vi "Protocol Main.vi"() -> ()   [LabVIEW 2014]
doc: "Diese Vorlage beschreibt das Design \"Handler für Nachrichten-Queues\".\n\nDie Schleife zur Ereignisbehandlung erzeugt Nachrichten basierend auf Benutzereingaben.\n\nDie Schleife zur Nachrichtenbehandlung verarbeitet Nachrichten, die von der Ereignisschleife oder anderen Nachrichten erzeugt wurden. Die Nachrichten sind String-Werte. Neue Nachrichten können also einfach der Case-Struktur der Nachrichtenschleife hinzugefügt werden. Der Nachrichten-Cluster kann auch einen optionalen Wert für Nachrichtendaten enthalten. Dabei handelt es sich um einen Variant, der in beliebige nachrichtenspezifische Daten umgewandelt werden kann."
uses:
  controls/ProtocolT.ctl
  controls/ProtocolEntry.ctl
  controls/MyQH UI Data.ctl
  support/Message Queue/Enqueue Message (Single).vi
  support/Message Queue/Enqueue Message (Array).vi
  <vilib>/Utility/error.llb/Error Cluster From Error Code.vi
  <vilib>/ErrorRing/Error Ring.xnode
  support/Message Queue/MyQH Message Queue.lvlib
  support/User Event - Stop/MyQH User Event - Stop.lvlib
panel:
  in  "Load":bool
  in  "Save":bool
  in  "ProtocolT":T1 {"Zeitstempel" format=" %<%X %x>T"}
  out "Anzeige <Ersetzen>":string
  in  "Remove Entry":bool
  in  "Add Entry":bool
  in  "Beenden":bool
  # "Titel"
  # "Eintrag"
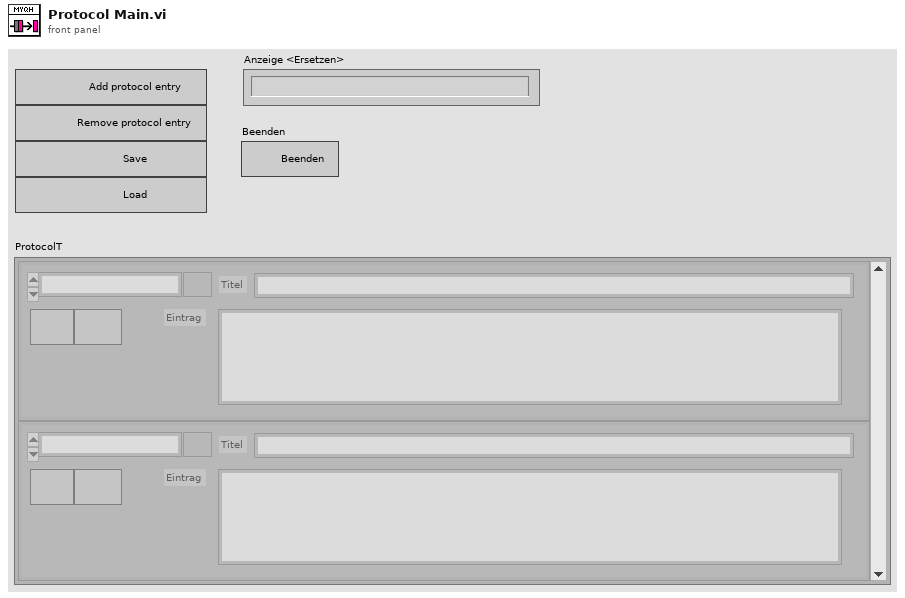
[diagram p1: front panel]
types:
  T1 = typedef "ProtocolT.ctl" = T2[]
  T2 = typedef "ProtocolEntry.ctl" = cluster{"Zeitstempel":timestamp, "String":string, "Abbrechen-Schaltfläche":bool, "Optionen-Schaltfläche":bool, "String 2":string}
  T3 = typedef "MyQH UI Data.ctl" = cluster{"Boolesch <Ersetzen>":bool, "String <Ersetzen>":string, "Numerisch <Ersetzen>":dbl, "Etwas tun (Ref.)":refnum<vi>, "Etwas anderes tun (Ref.)":refnum<vi>, "Datenanzeige (Ref.)":refnum<vi>, "Beenden-Schaltfl. (Ref.)":refnum<vi>, "Cluster":cluster{"VI Referenz":refnum<vi>}, "Arr Referenz":refnum<vi>, "Cluster Referenz":refnum<vi>, "ProtocolT":T1, "ProtocolEntryT":T2}
  T4 = cluster{"Status":bool, "Code":i32, "Quelle":string}
  T5 = typedef "MyQH Message Queue.lvlib/All Message Queues.ctl" = cluster{"UI":refnum<queue>}
  T6 = enum16{"big-endian, network order", "native, host order", "little-endian"}
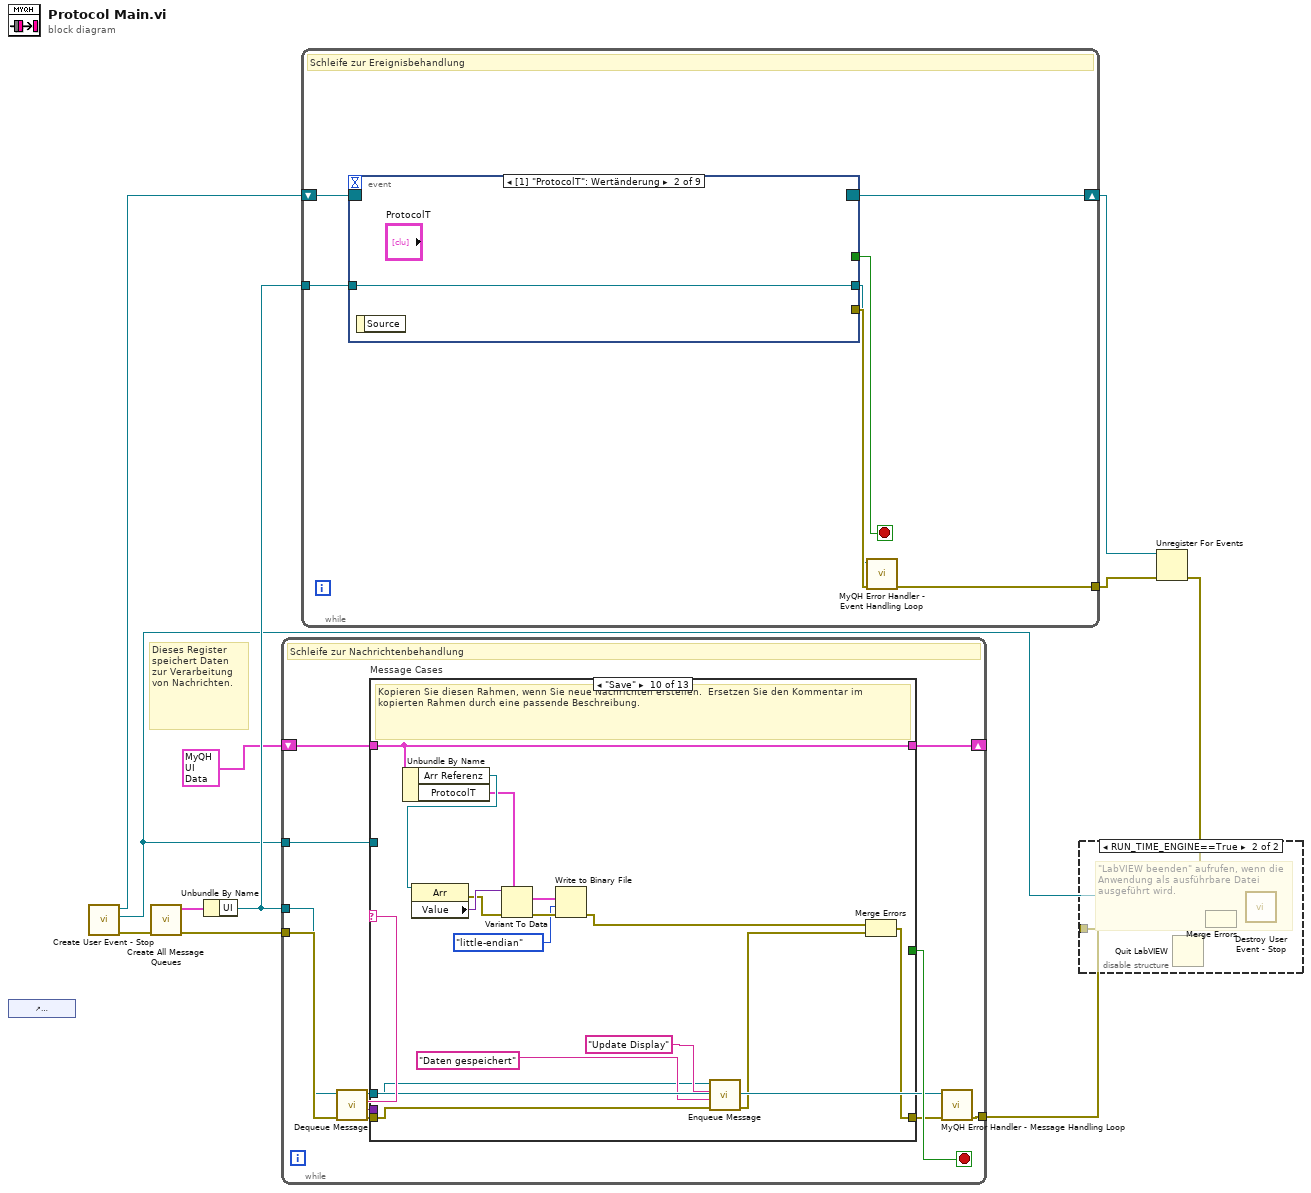
[diagram p0: block diagram]
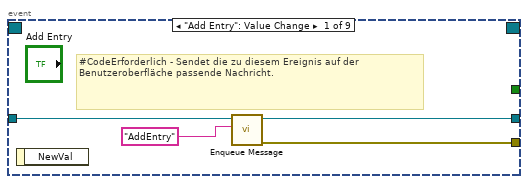
[diagram p3: hidden frame]
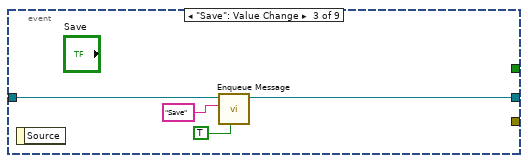
[diagram p4: hidden frame]
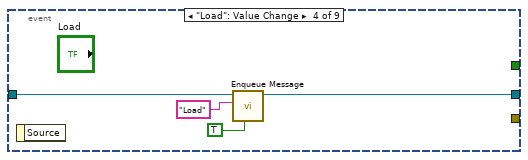
[diagram p5: hidden frame]
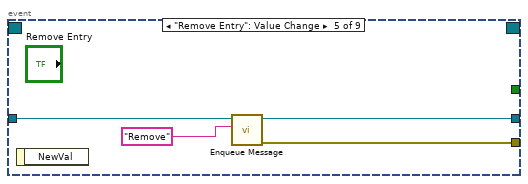
[diagram p6: hidden frame]
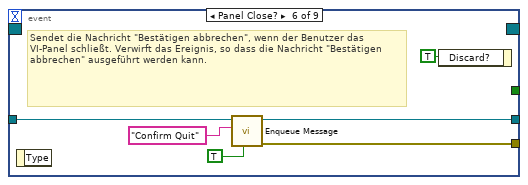
[diagram p7: hidden frame]
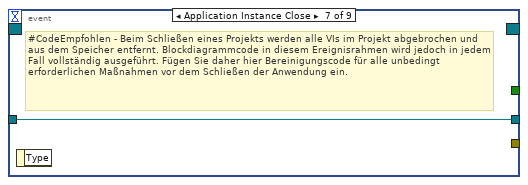
[diagram p8: hidden frame]
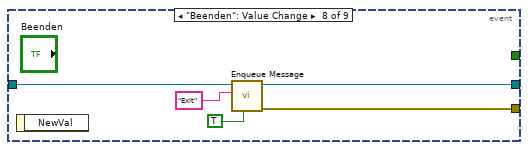
[diagram p9: hidden frame]
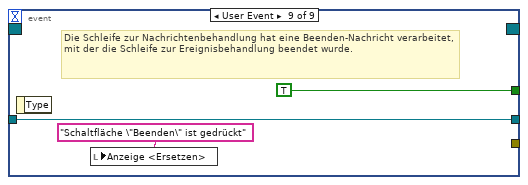
[diagram p10: hidden frame]
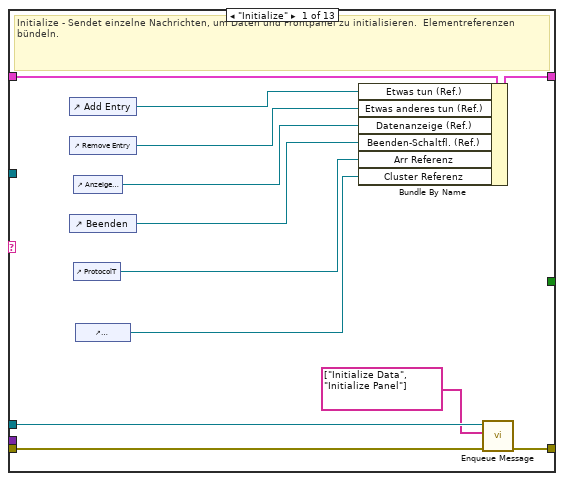
[diagram p11: hidden frame]
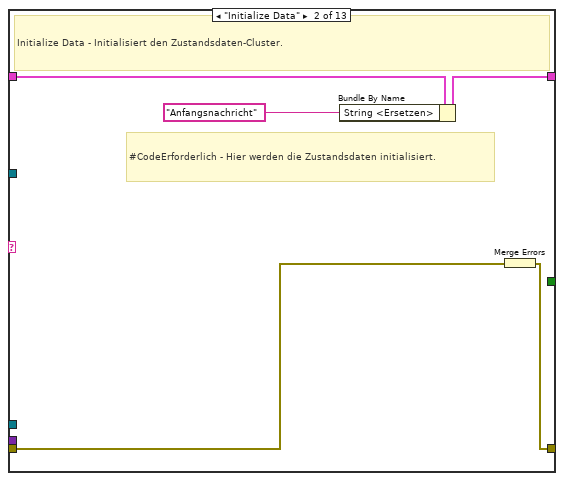
[diagram p12: hidden frame]
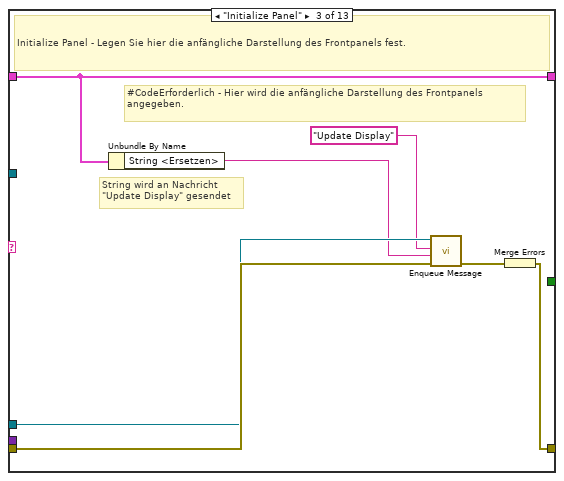
[diagram p13: hidden frame]
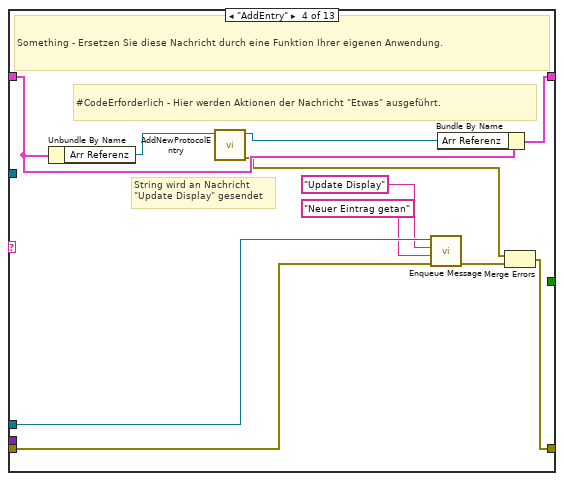
[diagram p14: hidden frame]
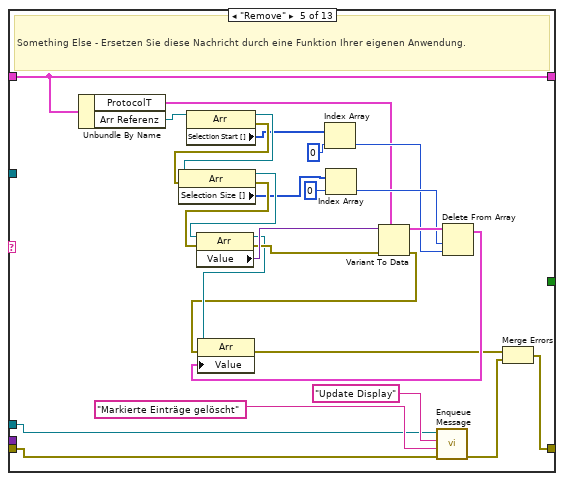
[diagram p15: hidden frame]
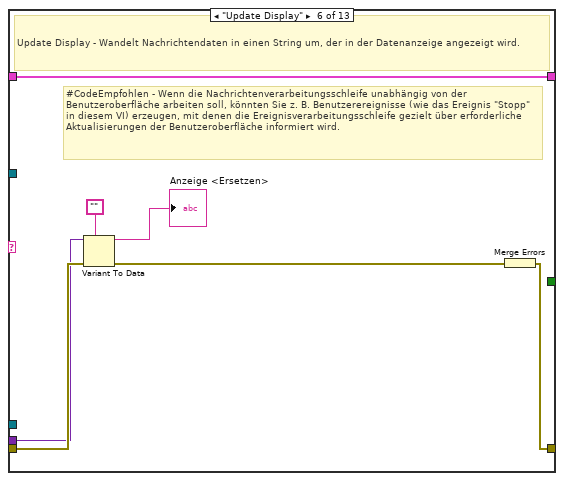
[diagram p16: hidden frame]
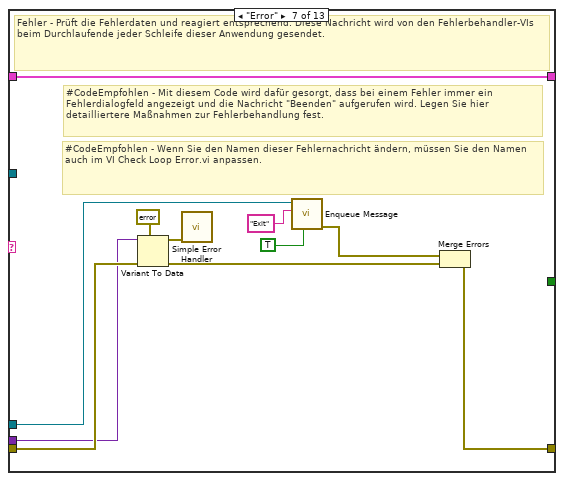
[diagram p17: hidden frame]
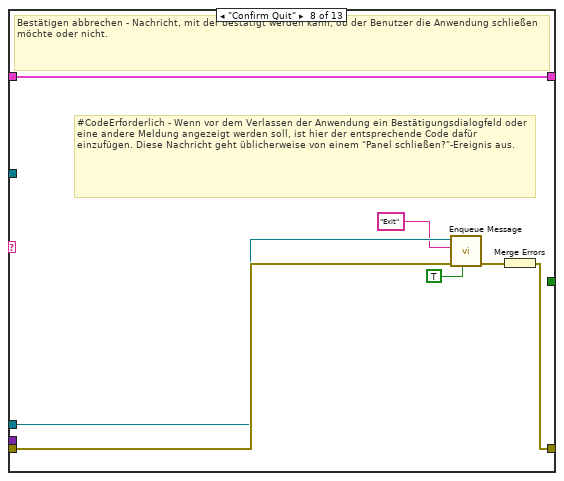
[diagram p18: hidden frame]
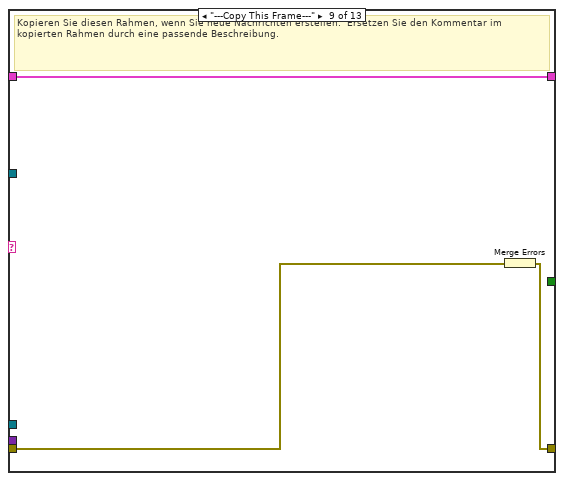
[diagram p19: hidden frame]
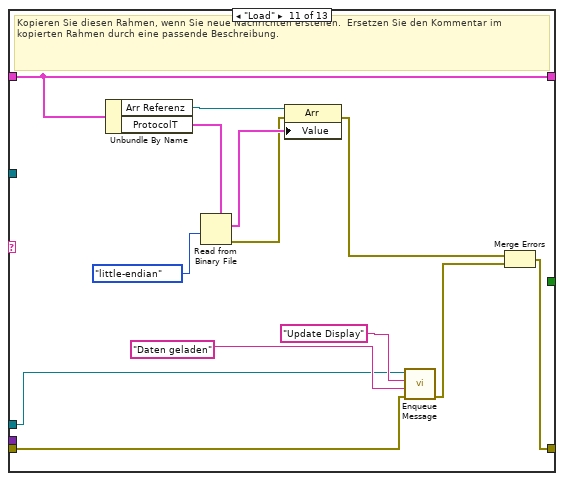
[diagram p20: hidden frame]
diagram:
  # "Dieses Register speichert Daten zur Verarbeitung von Nachrichten."
  n1 = control-ref of="Abbrechen-Schaltfläche"() -> ()  [unwired: 1 out]
  n2 = call "Create User Event - Stop.vi"() -> ("error out"=w8:T4, "Benutzerereignis - Stopp"=w6:refnum<user-event>, "Stoppereignisregistrierung (Referenz)"=w9:refnum<event-registration>)  [unwired: 9 in]
  n3 = call "Create All Message Queues.vi"("error in (no error)"=w8) -> ("error out"=w13:T4, "Nachrichten-Queues (Ausgang)"=w12:T5)  [unwired: 9 in]
  n4 = Unbundle By Name(w12) -> ("UI"=w10:refnum<queue>)
  n5 = while {
    tunnel: w10 -> [w17]
    shift-right: [w24] -> _
    shift-left: T3 {"Boolesch <Ersetzen>"=FALSE, "String <Ersetzen>"="", "Numerisch <Ersetzen>"=0.0, "Etwas tun (Ref.)"=refnum, "Etwas anderes tun (Ref.)"=refnum, "Datenanzeige (Ref.)"=refnum, "Beenden-Schaltfl. (Ref.)"=refnum, "Cluster"={"VI Referenz"=refnum}, "Arr Referenz"=refnum, "Cluster Referenz"=refnum, "ProtocolT"=[], "ProtocolEntryT"={"Zeitstempel"=timestamp(0 s since 1904-01-01), "String"="", "Abbrechen-Schaltfläche"=FALSE, "Optionen-Schaltfläche"=FALSE, "String 2"=""}} ("Data Cluster") -> [w25]
    tunnel: w6 -> [w22]
    tunnel: w13 -> [w21]
    tunnel: [w15] -> w11
    stop <- w23 stop-if-true
    # "Schleife zur Nachrichtenbehandlung"
    n6 = call "Dequeue Message.vi"("error in (no error)"=w21, "Nachrichten-Queue"=w17) -> ("error out"=w20:T4, "Nachrichtendaten"=w18:variant, "Nachricht"=w19:string, "Nachrichten-Queue (Kopie)"=w16:refnum<queue>)  [unwired: 6 in]
    n7 = case "Message Cases" shown="\"Save\"" w19 {
      selector: w19 -> [_ _ _ _ _ _ _ _ _ _ _ _ w151]
      tunnel: w16 -> [w35 _ w46 w57 w63 _ w96 w107 _ w116 w132 w150 _]
      tunnel: w20 -> [w36 w42 w47 w59 w62 w91 w104 w111 w114 w117 w130 w145 _]
      tunnel: [w37 w38 w48 w60 w86 w92 w97 w109 w112 w129 w142 w146 w152] -> w14
      tunnel: w25 -> [w34 w41 w49 w52 w67 w93 w103 w110 w113 w128 w140 w149 w153]
      tunnel: [w33 w40 w49 w51 w67 w93 w103 w110 w113 w128 w140 w149 w153] -> w24
      tunnel: [_ _ _ _ _ _ _ _ _ _ _ TRUE _] -> w23
      tunnel: w18 -> [_ _ _ _ _ w90 w102 _ _ _ _ _ _]
      tunnel: w22 -> [_ _ _ _ _ _ _ _ _ _ _ w144 _]
      frame "Initialize" {
        # "Initialize - Sendet einzelne Nachrichten, um Daten und Frontpanel zu initialisieren.  Elementreferenzen bündeln."
        n8 = control-ref of="Add Entry"() -> (w32:refnum<vi>)
        n9 = control-ref of="Remove Entry"() -> (w31:refnum<vi>)
        n10 = control-ref of="Beenden"() -> (w29:refnum<vi>)
        n11 = control-ref of="Anzeige <Ersetzen>"() -> (w30:refnum<vi>)
        n12 = control-ref of="ProtocolT"() -> (w27:refnum<vi>)
        n13 = control-ref of="ProtocolEntryT"() -> (w26:refnum<vi>)
        n14 = Bundle By Name(cluster=w34, "Etwas tun (Ref.)"=w32, "Etwas anderes tun (Ref.)"=w31, "Datenanzeige (Ref.)"=w30, "Beenden-Schaltfl. (Ref.)"=w29, "Arr Referenz"=w27, "Cluster Referenz"=w26) -> (w33:T3)
        n15 = call-poly "Enqueue Message.vi"("error in (no error)"=w36, "Nachrichten-Array"=string[] ["Initialize Data", "Initialize Panel"], "Nachrichten-Queue"=w35) -> ("error out"=w37:T4)  [unwired: 7 in, 1 out]
      }
      frame "Initialize Data" {
        # "#CodeErforderlich - Hier werden die Zustandsdaten initialisiert."
        # "Initialize Data - Initialisiert den Zustandsdaten-Cluster."
        n16 = Bundle By Name(cluster=w41, "String <Ersetzen>"="Anfangsnachricht" ("Initial Message")) -> (w40:T3)
        n17 = Merge Errors(w42) -> (w38:errorcluster)
      }
      frame "Initialize Panel" {
        # "String wird an Nachricht\n\"Update Display\" gesendet"
        # "#CodeErforderlich - Hier wird die anfängliche Darstellung des Frontpanels angegeben."
        # "Initialize Panel - Legen Sie hier die anfängliche Darstellung des Frontpanels fest."
        n18 = Unbundle By Name(w49) -> ("String <Ersetzen>"=w43:string)
        n19 = call-poly "Enqueue Message.vi"("error in (no error)"=w47, "Nachrichtendaten"=w43, "Nachricht"="Update Display" ("Message"), "Nachrichten-Queue"=w46) -> ("error out"=w45:T4)  [unwired: 6 in, 1 out]
        n20 = Merge Errors(w45) -> (w48:errorcluster)
      }
      frame "AddEntry" {
        # "String wird an Nachricht\n\"Update Display\" gesendet"
        # "#CodeErforderlich - Hier werden Aktionen der Nachricht \"Etwas\" ausgeführt."
        # "Something - Ersetzen Sie diese Nachricht durch eine Funktion Ihrer eigenen Anwendung."
        n21 = Unbundle By Name(w52) -> ("Arr Referenz"=w54:refnum<vi>)
        n22 = call "AddNewProtocolEntry.vi"("Array (Eingang)"=w54) -> ("Fehler (Ausgang)"=w50:errorcluster, "Referenz (Ausgang)"=w53:refnum<vi>)  [unwired: 9 in]
        n23 = call-poly "Enqueue Message.vi"("error in (no error)"=w59, "Nachrichtendaten"="Neuer Eintrag getan" ("\"Do Something\" button pressed"), "Nachricht"="Update Display" ("Message"), "Nachrichten-Queue"=w57) -> ("error out"=w58:T4)  [unwired: 6 in, 1 out]
        n24 = Bundle By Name(cluster=w52, "Arr Referenz"=w53) -> (w51:T3)
        n25 = Merge Errors(w50, w58) -> (w60:errorcluster)
      }
      frame "Remove" {
        # "Something Else - Ersetzen Sie diese Nachricht durch eine Funktion Ihrer eigenen Anwendung."
        n26 = Unbundle By Name(w67) -> ("ProtocolT"=w66:T1, "Arr Referenz"=w85:refnum<vi>)
        n27 = property class="Arr"(reference=w85) -> (reference out=w83:refnum<vi>, error out=w84:errorcluster, "Selection Start []"=w77:u32[])  [unwired: 1 in]
        n28 = property class="Arr"(reference=w83, error in=w84) -> (reference out=w80:refnum<vi>, error out=w79:errorcluster, "Selection Size []"=w74:u32[])
        n29 = property class="Arr"(reference=w80, error in=w79) -> (reference out=w70:refnum<vi>, error out=w81:errorcluster, "Value"=w82:variant)
        n30 = Index Array(array=w77, index=0 ("Index")) -> (element=w72:u32)
        n31 = Index Array(array=w74, index=0 ("Index")) -> (element=w73:u32)
        n32 = Variant To Data(error in=w81, type=w66, Variant=w82) -> (data=w78:T1, error out=w69:errorcluster)
        n33 = call-poly "Enqueue Message.vi"("error in (no error)"=w62, "Nachrichtendaten"="Markierte Einträge gelöscht" ("\"Do Something\" button pressed"), "Nachricht"="Update Display" ("Message"), "Nachrichten-Queue"=w63) -> ("error out"=w61:T4)  [unwired: 6 in, 1 out]
        n34 = Delete From Array(array=w78, length=w73, index=w72) -> (array with subset deleted=w71:T1)  [unwired: 1 out]
        n35 = property class="Arr"(reference=w70, error in=w69, "Value"=w71) -> (error out=w68:errorcluster)  [unwired: 1 out]
        n36 = Merge Errors(w68, w61) -> (w86:errorcluster)
      }
      frame "Update Display" {
        # "#CodeEmpfohlen - Wenn die Nachrichtenverarbeitungsschleife unabhängig von der Benutzeroberfläche arbeiten soll, könnten Sie z. B. Benutzerereignisse (wie das Ereignis \"Stopp\" in diesem VI) erzeugen, mit denen die Ereignisverarbeitungsschleife gezielt über erforderliche Aktualisierungen der Benutzeroberfläche informiert wird."
        # "Update Display - Wandelt Nachrichtendaten in einen String um, der in der Datenanzeige angezeigt wird."
        n37 = Variant To Data(error in=w91, type="", Variant=w90) -> (data=→"Anzeige <Ersetzen>":string, error out=w88:errorcluster)
        n38 = Merge Errors(w88) -> (w92:errorcluster)
      }
      frame "Error" {
        # "#CodeEmpfohlen - Wenn Sie den Namen dieser Fehlernachricht ändern, müssen Sie den Namen auch im VI Check Loop Error.vi anpassen."
        # "#CodeEmpfohlen - Mit diesem Code wird dafür gesorgt, dass bei einem Fehler immer ein Fehlerdialogfeld angezeigt und die Nachricht \"Beenden\" aufgerufen wird. Legen Sie hier detailliertere Maßnahmen zur Fehlerbehandlung fest."
        # "Fehler - Prüft die Fehlerdaten und reagiert entsprechend. Diese Nachricht wird von den Fehlerbehandler-VIs beim Durchlaufende jeder Schleife dieser Anwendung gesendet."
        n39 = Variant To Data(error in=w104, type=errorcluster {"status"=FALSE, "code"=0, "source"=""} ("error constant"), Variant=w102) -> (data=w100:errorcluster, error out=w99:errorcluster)
        n40 = call <vilib>:"Simple Error Handler.vi"("error in (no error)"=w100) -> ()  [unwired: 4 in, 5 out]
        n41 = call-poly "Enqueue Message.vi"("Nachricht mit Priorität? (F)"=TRUE ("Priority Message? (F)"), "Nachricht"="Exit", "Nachrichten-Queue"=w96) -> ("error out"=w98:T4)  [unwired: 7 in, 1 out]
        n42 = Merge Errors(w98, w99) -> (w97:errorcluster)
      }
      frame "Confirm Quit" {
        # "#CodeErforderlich - Wenn vor dem Verlassen der Anwendung ein Bestätigungsdialogfeld oder eine andere Meldung angezeigt werden soll, ist hier der entsprechende Code dafür einzufügen. Diese Nachricht geht üblicherweise von einem \"Panel schließen?\"-Ereignis aus."
        # "Bestätigen abbrechen - Nachricht, mit der bestätigt werden kann, ob der Benutzer die Anwendung schließen möchte oder nicht."
        n43 = call-poly "Enqueue Message.vi"("Nachricht mit Priorität? (F)"=TRUE ("Priority Message? (F)"), "error in (no error)"=w111, "Nachricht"="Exit" ("Message"), "Nachrichten-Queue"=w107) -> ("error out"=w108:T4)  [unwired: 6 in, 1 out]
        n44 = Merge Errors(w108) -> (w109:errorcluster)
      }
      frame "---Copy This Frame---" {
        # "Kopieren Sie diesen Rahmen, wenn Sie neue Nachrichten erstellen.  Ersetzen Sie den Kommentar im kopierten Rahmen durch eine passende Beschreibung."
        n45 = Merge Errors(w114) -> (w112:errorcluster)
      }
      frame "Save" {
        # "Kopieren Sie diesen Rahmen, wenn Sie neue Nachrichten erstellen.  Ersetzen Sie den Kommentar im kopierten Rahmen durch eine passende Beschreibung."
        n46 = Unbundle By Name(w128) -> ("Arr Referenz"=w127:refnum<vi>, "ProtocolT"=w120:T1)
        n47 = property class="Arr"(reference=w127) -> (error out=w125:errorcluster, "Value"=w126:variant)  [unwired: 1 in, 1 out]
        n48 = Variant To Data(error in=w125, type=w120, Variant=w126) -> (data=w124:T1, error out=w123:errorcluster)
        n49 = Write to Binary File(data=w124, error in=w123, 9:T6."little-endian" ("Byte-Reihenfolge (0:Big-Endian, Netzwerkreihenfolge)")) -> (error out=w121:errorcluster)  [unwired: 3 in, 2 out]
        n50 = call-poly "Enqueue Message.vi"("error in (no error)"=w117, "Nachrichtendaten"="Daten gespeichert" ("\"Do Something\" button pressed"), "Nachricht"="Update Display" ("Message"), "Nachrichten-Queue"=w116) -> ("error out"=w115:T4)  [unwired: 6 in, 1 out]
        n51 = Merge Errors(w121, w115) -> (w129:errorcluster)
      }
      frame "Load" {
        # "Kopieren Sie diesen Rahmen, wenn Sie neue Nachrichten erstellen.  Ersetzen Sie den Kommentar im kopierten Rahmen durch eine passende Beschreibung."
        n52 = Unbundle By Name(w140) -> ("Arr Referenz"=w139:refnum<vi>, "ProtocolT"=w135:T1)
        n53 = Read from Binary File(5:w135, 9:T6."little-endian" ("Byte-Reihenfolge (0:Big-Endian, Netzwerkreihenfolge)")) -> (0:w137:errorcluster, 2:w138:T1)  [unwired: 4 in, 2 out]
        n54 = property class="Arr"(reference=w139, error in=w137, "Value"=w138) -> (error out=w136:errorcluster)  [unwired: 1 out]
        n55 = call-poly "Enqueue Message.vi"("error in (no error)"=w130, "Nachrichtendaten"="Daten geladen" ("\"Do Something\" button pressed"), "Nachricht"="Update Display" ("Message"), "Nachrichten-Queue"=w132) -> ("error out"=w131:T4)  [unwired: 6 in, 1 out]
        n56 = Merge Errors(w136, w131) -> (w142:errorcluster)
      }
      frame "Exit" {
        # "Stoppt das VI."
        # "Nachrichten-Queue-Referenz wird freigegeben"
        # "#CodeErforderlich - Fügen Sie hier Bereinigungscode ein."
        # "Exit - Programm schließen"
        n57 = call "Fire User Event - Stop.vi"("Benutzerereignis - Stopp"=w144) -> ("error out"=w143:T4)  [unwired: 10 in]
        n58 = Release Queue(queue=w150, error in (no error)=w145) -> (error out=w147:errorcluster)  [unwired: 1 in, 2 out]
        n59 = Merge Errors(w143, w147) -> (w146:errorcluster)
      }
      frame Default {
        # "Der Case \"Standard\" wird nur ausgeführt, wenn eine Nachricht vorliegt, die in keinem anderen Case definiert ist.  Es wird ein Programmierfehler ausgegeben."
        n60 = xnode "Fehlerring"("Parameter 0"=w151) -> ("Fehler (Ausgang)"=w152:errorcluster)
      }
    }
    n61 = call "MyQH Error Handler - Message Handling Loop.vi"("error in (no error)"=w14, "Nachrichten-Queue"=w16) -> ("Fehler (Eingang, Kopie)"=w15:T4)  [unwired: 8 in, 1 out]
  }
  n62 = while {
    tunnel: w10 -> [w167]
    shift-right: [w165] -> w4
    shift-left: w9 -> [w166]
    tunnel: [w161] -> w1
    stop <- w163 stop-if-true
    # "Schleife zur Ereignisbehandlung"
    n63 = event shown="[1] \"ProtocolT\": Wertänderung" {
      selector: w166 -> [_ _ _ _ _ _ _ _ _]
      dyn-events: [_ _ _ _ _ _ _ _ _] -> w165
      timeout: _ -> [_ _ _ _ _ _ _ _ _]
      tunnel: [_ _ _ _ _ _ _ _ TRUE ("Discard?")] -> w163
      tunnel: w167 -> [w171 w172 w174 w178 w184 w189 w191 w196 w199]
      tunnel: [w168 _ _ _ w181 w188 _ w195 _] -> w164
      tunnel: [w170 w172 w173 w177 w183 w187 w191 w194 w199] -> w162
      event "Add Entry": Value Change {
        # "#CodeErforderlich - Sendet die zu diesem Ereignis auf der Benutzeroberfläche passende Nachricht."
        n64 = event-data() -> ()  [unwired: 1 in, 1 out]
        n65 = call-poly "Enqueue Message.vi"("Nachricht"="AddEntry" ("Message"), "Nachrichten-Queue"=w171) -> ("error out"=w168:T4, "Nachrichten-Queue (Kopie)"=w170:refnum<queue>)  [unwired: 8 in]
      }
      event Value Change {
        n66 = event-data() -> ()  [unwired: 1 in, 1 out]
      }
      event "Save": Value Change {
        n67 = event-data() -> ()  [unwired: 1 in, 1 out]
        n68 = call-poly "Enqueue Message.vi"("Nachricht mit Priorität? (F)"=TRUE ("Priority Message? (F)"), "Nachricht"="Save" ("Message"), "Nachrichten-Queue"=w174) -> ("Nachrichten-Queue (Kopie)"=w173:refnum<queue>)  [unwired: 7 in, 1 out]
      }
      event "Load": Value Change {
        n69 = event-data() -> ()  [unwired: 1 in, 1 out]
        n70 = call-poly "Enqueue Message.vi"("Nachricht mit Priorität? (F)"=TRUE ("Priority Message? (F)"), "Nachricht"="Load" ("Message"), "Nachrichten-Queue"=w178) -> ("Nachrichten-Queue (Kopie)"=w177:refnum<queue>)  [unwired: 7 in, 1 out]
      }
      event "Remove Entry": Value Change {
        n71 = event-data() -> ()  [unwired: 1 in, 1 out]
        n72 = call-poly "Enqueue Message.vi"("Nachricht"="Remove" ("Message"), "Nachrichten-Queue"=w184) -> ("error out"=w181:T4, "Nachrichten-Queue (Kopie)"=w183:refnum<queue>)  [unwired: 8 in]
      }
      event Panel Close? {
        # "Sendet die Nachricht \"Bestätigen abbrechen\", wenn der Benutzer das VI-Panel schließt. Verwirft das Ereignis, so dass die Nachricht \"Bestätigen abbrechen\" ausgeführt werden kann."
        n73 = event-data() -> ()  [unwired: 1 in, 1 out]
        n74 = call-poly "Enqueue Message.vi"("Nachricht mit Priorität? (F)"=TRUE ("Priority Message? (F)"), "Nachricht"="Confirm Quit" ("Message"), "Nachrichten-Queue"=w189) -> ("error out"=w188:T4, "Nachrichten-Queue (Kopie)"=w187:refnum<queue>)  [unwired: 7 in]
        n75 = event-data("Discard?"=TRUE) -> ()  [unwired: 1 in, 1 out]
      }
      event Application Instance Close {
        # "#CodeEmpfohlen - Beim Schließen eines Projekts werden alle VIs im Projekt abgebrochen und aus dem Speicher entfernt. Blockdiagrammcode in diesem Ereignisrahmen wird jedoch in jedem Fall vollständig ausgeführt. Fügen Sie daher hier Bereinigungscode für alle unbedingt erforderlichen Maßnahmen vor dem Schließen der Anwendung ein."
        n76 = event-data() -> ()  [unwired: 1 in, 1 out]
      }
      event "Beenden": Value Change {
        n77 = event-data() -> ()  [unwired: 1 in, 1 out]
        n78 = call-poly "Enqueue Message.vi"("Nachricht mit Priorität? (F)"=TRUE ("Priority Message? (F)"), "Nachricht"="Exit" ("Message"), "Nachrichten-Queue"=w196) -> ("error out"=w195:T4, "Nachrichten-Queue (Kopie)"=w194:refnum<queue>)  [unwired: 7 in]
      }
      event User Event {
        # "Die Schleife zur Nachrichtenbehandlung hat eine Beenden-Nachricht verarbeitet, mit der die Schleife zur Ereignisbehandlung beendet wurde."
        n79 = event-data() -> ()  [unwired: 1 in, 1 out]
        n80 = local write "Anzeige <Ersetzen>"("Schaltfläche \"Beenden\" ist gedrückt" ("VI Stopped")) -> ()
      }
    }
    n81 = call "MyQH Error Handler - Event Handling Loop.vi"("error in (no error)"=w164, "Nachrichten-Queue"=w162) -> ("Fehler (Eingang, Kopie)"=w161:T4)  [unwired: 8 in, 1 out]
  }
  n82 = Unregister For Events(event registration refnum=w4, error in=w1) -> (error out=w5:errorcluster)
  n83 = Merge Errors(w5, w11) -> (w7:errorcluster)
  n84 = call "Destroy User Event - Stop.vi"("error in (no error)"=w7, "Benutzerereignis - Stopp"=w6) -> ("error out"=w2:T4)  [unwired: 9 in]
  n85 = disable-structure shown="RUN_TIME_ENGINE==True" {
    disable-tunnel: w2 -> [_ _]
    frame condition #0 (active) {
    }
    frame condition #1 {
      # "\"LabVIEW beenden\" aufrufen, wenn die Anwendung als ausführbare Datei ausgeführt wird."
      n86 = Quit LabVIEW() -> ()  [unwired: 1 in]
    }
  }
